vi "joint.vi"(0 "Attributes":T4, 2 "type":T2, 3 "Name":string="joint_name") -> (4 "Joint":T1={"Joint Name"="left_wheel_hinge", "type"=enum."revolute", "urdf "="", "Links"=[]})   [LabVIEW 2010]
uses:
  JointTypes.ctl
  LINK.ctl
  JOINT.ctl
  JointAttributes.ctl
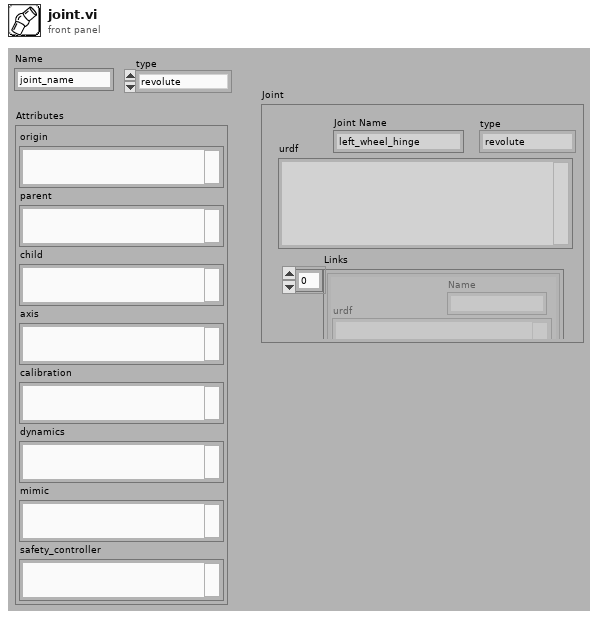
[diagram p1: front panel]
types:
  T1 = typedef "JOINT.ctl" = cluster{"Joint Name":string, "type":T2, "urdf ":string, "Links":T3[]}
  T2 = typedef "JointTypes.ctl" = enum16{"revolute", "continuous", "prismatic", "fixed", "floating", "planar"}
  T3 = typedef "LINK.ctl" = cluster{"Name":string, "urdf":string}
  T4 = typedef "JointAttributes.ctl" = cluster{"origin":string, "parent":string, "child":string, "axis":string, "calibration":string, "dynamics":string, "mimic":string, "safety_controller":string}
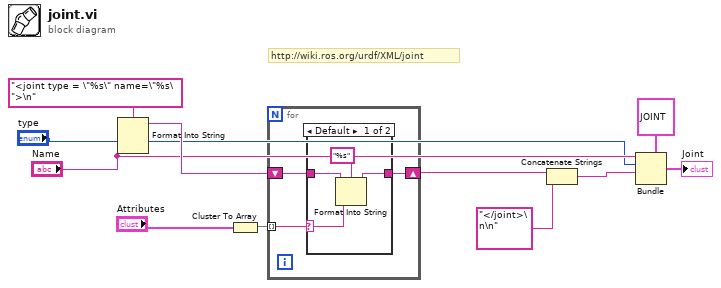
[diagram p0: block diagram]
diagram:
  # "http://wiki.ros.org/urdf/XML/joint"
  n1 = Format Into String(format string="<joint type = \"%s\" name=\"%s\">\n", "type", "Name") -> (resulting string=w11:string)  [unwired: 2 in, 1 out]
  n2 = Cluster To Array(cluster="Attributes") -> (array=w7:string[])
  n3 = for {
    shift-right: [w14] -> w9
    shift-left: w11 -> [w13]
    tunnel: w7 -> [w12] mode=indexing
    n4 = case shown="Default" w12 {
      selector: w12 -> [w16 _]
      tunnel: [w15 w19] -> w14
      tunnel: w13 -> [w18 w19]
      frame Default {
        n5 = Format Into String(format string="%s", initial string=w18, w16) -> (resulting string=w15:string)  [unwired: 1 in, 1 out]
      }
      frame "" {
      }
    }
  }
  n6 = Concatenate Strings(w9, "</joint>\n\n") -> (w5:string)
  n7 = Bundle(cluster=T1 {"Joint Name"="left_wheel_hinge", "type"=enum."revolute", "urdf "="", "Links"=[]} ("Joint"), "Joint Name"="Name", "type"="type", "urdf"=w5) -> (→"Joint":T1)  [unwired: 1 in]
